vi "TDMS Init.vi"(8 "error in (no error)":errorcluster, 11 "tdms file":refnum<k34>) -> (0 "error out":errorcluster, 3 "tdms file out":refnum<k34>)   [LabVIEW 2014]
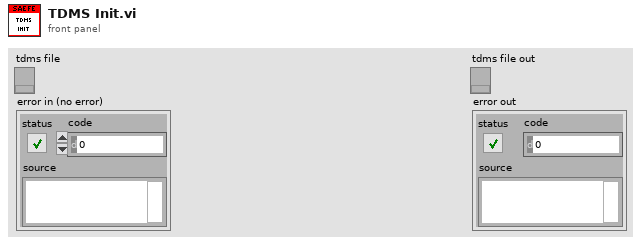
[diagram p1: front panel]
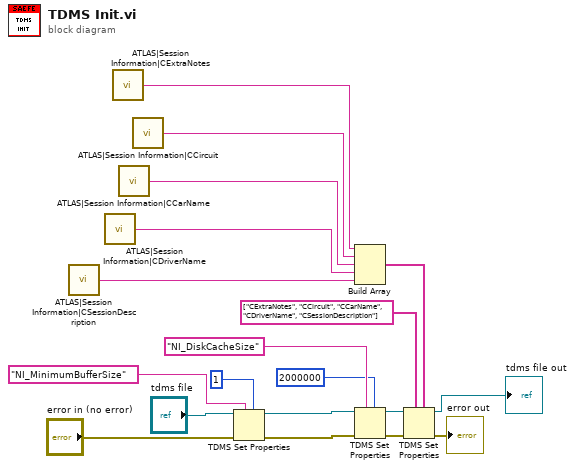
[diagram p0: block diagram]
diagram:
  n1 = call "ATLAS|Session Information|CSessionDescription"() -> ("Value"=w5:string)
  n2 = call "ATLAS|Session Information|CDriverName"() -> ("Value"=w6:string)
  n3 = call "ATLAS|Session Information|CExtraNotes"() -> ("Value"=w9:string)
  n4 = call "ATLAS|Session Information|CCarName"() -> ("Value"=w7:string)
  n5 = call "ATLAS|Session Information|CCircuit"() -> ("Value"=w8:string)
  n6 = TDMS Set Properties(5:u32 1, 7:"NI_MinimumBufferSize", 8:"error in (no error)", 11:"tdms file") -> (0:w16:errorcluster, 3:w17:refnum<k34>)  [unwired: 2 in, 2 out]
  n7 = Build Array(w9, w8, w7, w6, w5) -> (w4:string[])
  n8 = TDMS Set Properties(5:u32 2000000, 7:"NI_DiskCacheSize", 8:w16, 11:w17) -> (0:w10:errorcluster, 3:w11:refnum<k34>)  [unwired: 2 in, 2 out]
  n9 = TDMS Set Properties(5:w4, 7:string[] ["CExtraNotes", "CCircuit", "CCarName", "CDriverName", "CSessionDescription"] ("property names"), 8:w10, 11:w11) -> (0:→"error out":errorcluster, 3:→"tdms file out":refnum<k34>)  [unwired: 2 in, 2 out]
